vi "Dodawanie punktów z listy współrzędnych.vi"(6 "Lista współrzędnych":string[][](array[string]), 9 "Właściwości punktów z listy":T1, 10 "Długość piksela w metrach":dbl, 11 "Mapa terenu":picture) -> (3 "Mapa z wprowadzonym punktem":picture)   [LabVIEW 2015, in "Biblioteka moduł map v3.lvlib" / "Obsługa grafiki mapy.lvlib"]
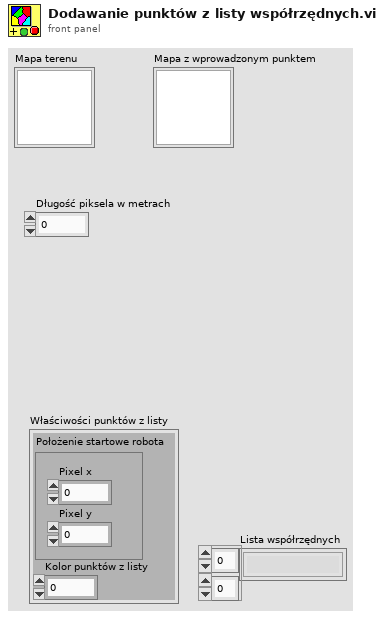
[diagram p1: front panel]
types:
  T1 = cluster{"Kolor punktów z listy":u32, "Położenie startowe robota":cluster{"Pixel x":i16, "Pixel y":i16}}
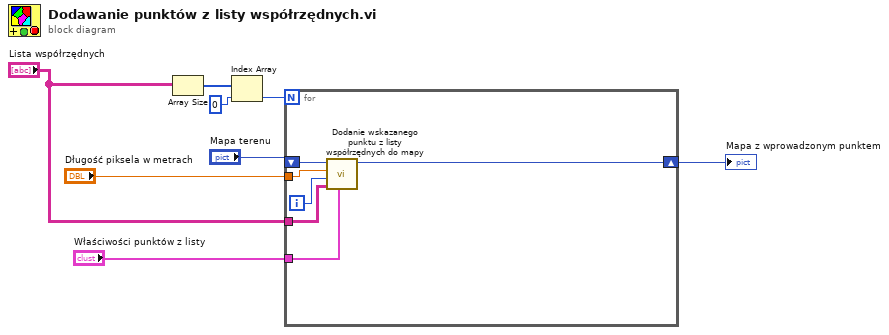
[diagram p0: block diagram]
diagram:
  n1 = Array Size(array="Lista współrzędnych") -> (size(s)=w7:i32[])
  n2 = Index Array(array=w7, index=0) -> (element=w6:i32)
  n3 = for {
    N: w6 -> [_]
    tunnel: "Lista współrzędnych" -> [w10]
    shift-right: [w14] -> w4
    shift-left: "Mapa terenu" -> [w11]
    tunnel: "Długość piksela w metrach" -> [w13]
    tunnel: "Właściwości punktów z listy" -> [w12]
    i -> [w9]
    n4 = call "Dodanie wskazanego punktu z listy współrzędnych do mapy.vi"("Właściwości punktów z listy"=w12, "Lista współrzędnych"=w10, "Nr punktu"=w9, "Długość piksela w metrach"=w13, "Mapa terenu"=w11) -> ("Mapa z wprowadzonym punktem"=w14:picture)  [unwired: 6 in]
  }
  "Mapa z wprowadzonym punktem" <- w4
